vi "Is IO Enable.vi"(8 "error in (no error)":errorcluster, 11 "channel":u8) -> (0 "error out":errorcluster, 3 "function return":u8)   [LabVIEW 2021, in "vmmsolib.lvlib"]
doc: "DLL_API unsigned char WINAPI IsIOEnable(unsigned char channel);"
uses:
  vmmsolib.lvlib
  vmmso.dll
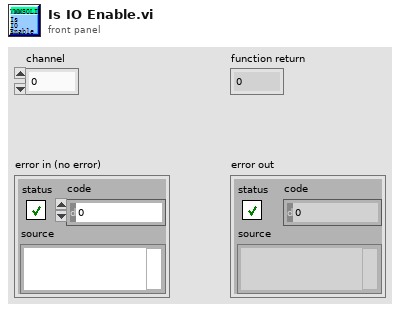
[diagram p1: front panel]
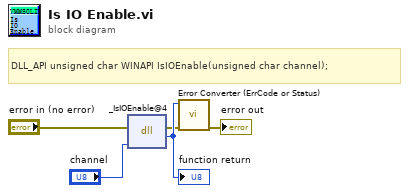
[diagram p0: block diagram]
diagram:
  # "DLL_API unsigned char WINAPI IsIOEnable(unsigned char channel);"
  n1 = dll-call lib="D:/VmMsoSDK/demo-Labview/2021/vmmsolib/vmmso.*" fn="_IsIOEnable@4"(error in="error in (no error)", "channel"="channel") -> (error out=w2:errorcluster, w5:u8)  [unwired: 3 in, 1 out]
  "function return" <- w5
  n2 = call "Error Converter (ErrCode or Status).vi"("error in (no error)"=w2, "error code"=w5) -> ("error out"=→"error out":errorcluster)  [unwired: 9 in]
